vi "Run Test Suite.vi"(8 "error in (no error)":errorcluster, 11 "Execution UI In":refnum<class "Execution UI.lvclass">) -> (0 "error out":errorcluster, 3 "Execution UI Out":refnum<class "Execution UI.lvclass">)   [LabVIEW 2020, in "Execution UI.lvclass"]
uses:
  Execution UI.lvclass
  Test Runner/Test Runner.lvclass
  Helper Classes/Test Result Tree/Test Result Tree.lvclass
  Helper Classes/Result Table/Result Table/Result Table.lvclass
  Report Generator/Report Generator.lvclass
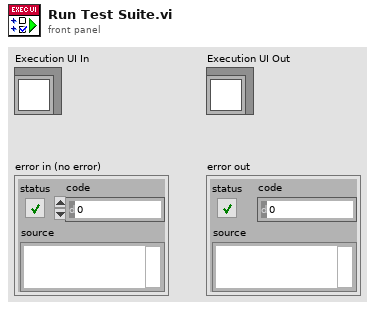
[diagram p1: front panel]
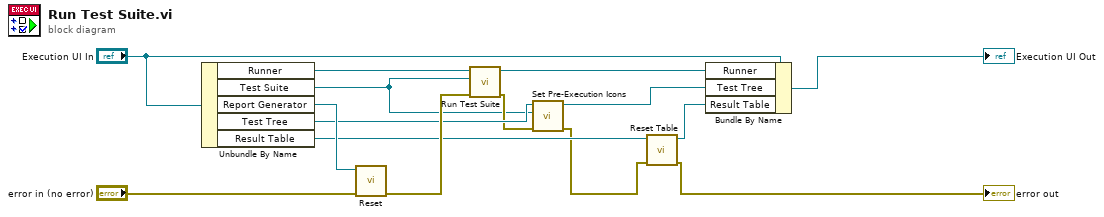
[diagram p0: block diagram]
diagram:
  n1 = Unbundle By Name("Execution UI In") -> ("Runner"=w12:refnum<class "Test Runner.lvclass">, "Test Suite"=w1:refnum<class "LUnit Test Suite.lvclass">, "Report Generator"=w13:refnum<class "Report Generator.lvclass">, "Test Tree"=w7:refnum<class "Test Result Tree.lvclass">, "Result Table"=w5:refnum<class "Result Table.lvclass">)
  n2 = call "Reset.vi"("error in (no error)"="error in (no error)", "Report Generator In"=w13) -> ("error out"=w14:errorcluster)  [unwired: 8 in, 1 out]
  n3 = call "Run Test Suite.vi"("error in (no error)"=w14, "Test Suite In"=w1, "Test Runner In"=w12) -> ("error out"=w6:errorcluster, "Test Runner Out"=w9:refnum<class "Test Runner.lvclass">)  [unwired: 7 in]
  n4 = call "Set Pre-Execution Icons.vi"("error in (no error)"=w6, "Test Suite"=w1, "Test Tree In"=w7) -> ("error out"=w3:errorcluster, "Test Tree Out"=w8:refnum<class "Test Result Tree.lvclass">)  [unwired: 7 in]
  n5 = call "Reset Table.vi"("error in (no error)"=w3, "Result Table.lvclass"=w5) -> ("error out"=→"error out":errorcluster, "Result Table"=w4:refnum<class "Result Table.lvclass">)  [unwired: 8 in]
  n6 = Bundle By Name(cluster="Execution UI In", "Runner"=w9, "Test Tree"=w8, "Result Table"=w4) -> (→"Execution UI Out":refnum<class "Execution UI.lvclass">)
